vi "PH_Beckhoff_PP_PU.handle PSU DIs.vi"(0 "i ref in":refnum<vi>, 2 "Digital Input Values":T1, 3 "Changed Digital Inputs":i32[](array[numeric]), 5 "error in":errorcluster) -> (14 "i ref out":refnum<vi>, 19 "error out":errorcluster)   [LabVIEW 2014, in "PH_Beckhoff_PP_PU.lvlib"]
uses:
  PH_Beckhoff_PP_PU.lvlib
  PH_Beckhoff/PH_Beckhoff.Digital Inputs.ctl
  PH_Basics/PH_StatusHandler/PH_StatusHandler.lvlib
  PH_Basics/PH_Common/PH_Common.lvlib
  PH_Beckhoff/PH_Beckhoff.lvlib
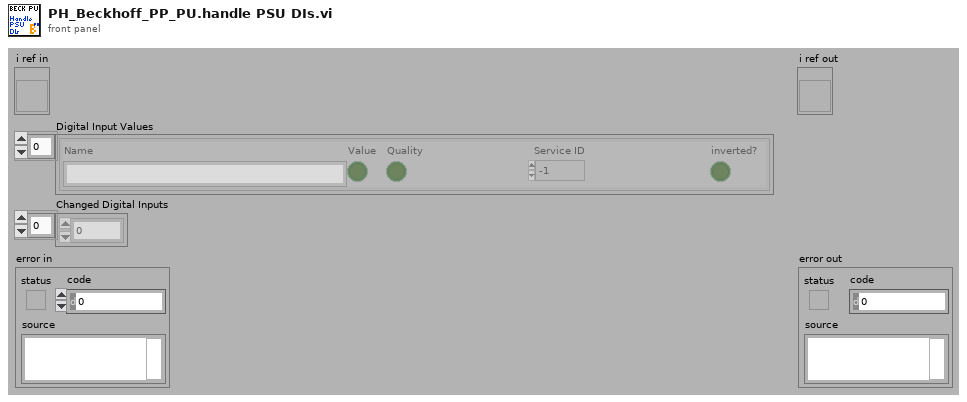
[diagram p1: front panel]
types:
  T1 = typedef "PH_Beckhoff.lvlib/PH_Beckhoff.Digital Inputs.ctl" = cluster{"Name":string, "Value":bool, "Quality":bool, "Service ID":i32, "inverted?":bool}[]
  T2 = typedef "PH_Beckhoff_PP_PU.lvlib/PH_Beckhoff_PP_PU.i attribute.ctl" = cluster{"HV Meas":cluster{"Input GUI Ref":refnum<vi>, "Voltage Service ID":i32, "Voltage [V]":dbl, "Quality":bool, "# in Data":i32}[], "Trigger":cluster{"Status":cluster{"GUI Ref":refnum<vi>, "Status Service ID":i32, "Status":T3}, "last shot:":cluster{"GUI Ref":refnum<vi>, "Service ID":i32, "Time":string}, "DIs":cluster{"triggered":cluster{"GUI Ref":refnum<vi>, "# in Data":i32}, "fired":cluster{"GUI Ref":refnum<vi>, "# in Data":i32}}, "GUI Ref Indicator":refnum<vi>}[], "RR":cluster{"Status":cluster{"GUI Ref":refnum<vi>, "Status Service ID":i32, "Status":T3}, "DIs":cluster{"closed":cluster{"GUI Ref":refnum<vi>, "# in Data":i32}, "open":cluster{"GUI Ref":refnum<vi>, "# in Data":i32}}, "Close":cluster{"GUI Ref":refnum<vi>, "# in Data":i32}, "GUI Ref Indicator":refnum<vi>}[], "Igni":cluster{"Status":cluster{"GUI Ref":refnum<vi>, "Status Service ID":i32, "Status":T3}, "DIs":cluster{"heating on":cluster{"GUI Ref":refnum<vi>, "# in Data":i32}, "water on":cluster{"GUI Ref":refnum<vi>, "# in Data":i32}}, "Device on":cluster{"GUI Ref":refnum<vi>, "# in Data":i32}, "GUI Ref Indicator":refnum<vi>}[], "PSU":cluster{"Status":cluster{"GUI Ref":refnum<vi>, "Status Service ID":i32, "Status":T3}, "Limit Service ID":i32, "DIs":cluster{"inhibit":cluster{"GUI Ref":refnum<vi>, "# in Data":i32}, "end of charge":cluster{"GUI Ref":refnum<vi>, "# in Data":i32}, "HV on":cluster{"GUI Ref":refnum<vi>, "# in Data":i32}, "overtemp":cluster{"GUI Ref":refnum<vi>, "# in Data":i32}, "interlock":cluster{"GUI Ref":refnum<vi>, "# in Data":i32}, "load fault":cluster{"GUI Ref":refnum<vi>, "# in Data":i32}, "sum fault":cluster{"GUI Ref":refnum<vi>, "# in Data":i32}, "HV off":cluster{"GUI Ref":refnum<vi>, "# in Data":i32}, "DC ok":cluster{"GUI Ref":refnum<vi>, "# in Data":i32}}, "AIs":cluster{"voltage":cluster{"GUI Ref":refnum<vi>, "# in Data":i32}, "current":cluster{"GUI Ref":refnum<vi>, "# in Data":i32}}, "DAs":cluster{"inhibit":cluster{"GUI Ref":refnum<vi>, "# in Data":i32}, "interlock":cluster{"GUI Ref":refnum<vi>, "# in Data":i32}, "HV on":cluster{"GUI Ref":refnum<vi>, "# in Data":i32}, "Reset":cluster{"GUI Ref":refnum<vi>, "# in Data":i32}}, "AAs":cluster{"Voltage to set":cluster{"GUI Ref":refnum<vi>, "# in Data":i32}}, "GUI Ref Indicator":refnum<vi>}[], "reconfigured":cluster{"?":bool, "GUI Ref":refnum<vi>}, "PU Rack Type":T4, "HV Meas Info":T5, "PSU Info":T6}
  T3 = typedef "PH_StatusHandler.lvlib/PH_StatusHandler.Status.ctl" = i16
  T4 = typedef "PH_Beckhoff_PP_PU.lvlib/PH_Beckhoff_PP_PU.PU Rack Type.ctl" = enum16{"no Info", "PA 19mm", "PA 45mm", "MA PU 1 and 2", "MA PU 3 and 4", "MA PU 5 and 6", "MA FR and PILC"}
  T5 = typedef "PH_Beckhoff_PP_PU.lvlib/PH_Beckhoff_PP_PU.HV Meas Info.ctl" = cluster{"Period Time [s]":dbl, "Subtractor 1 [Hz]":dbl, "Devider 1 [Hz/kV]":dbl, "Subtractor 2 [Hz]":dbl, "Devider 2 [Hz/kV]":dbl}
  T6 = typedef "PH_Beckhoff_PP_PU.lvlib/PH_Beckhoff_PP_PU.PSU Info.ctl" = cluster{"Limits 1 [V]":cluster{"Lower":dbl, "Upper":dbl}, "Limits 2 [V]":cluster{"Lower":dbl, "Upper":dbl}}
  T7 = cluster{"Status":cluster{"GUI Ref":refnum<vi>, "Status Service ID":i32, "Status":T3}, "Limit Service ID":i32, "DIs":cluster{"inhibit":cluster{"GUI Ref":refnum<vi>, "# in Data":i32}, "end of charge":cluster{"GUI Ref":refnum<vi>, "# in Data":i32}, "HV on":cluster{"GUI Ref":refnum<vi>, "# in Data":i32}, "overtemp":cluster{"GUI Ref":refnum<vi>, "# in Data":i32}, "interlock":cluster{"GUI Ref":refnum<vi>, "# in Data":i32}, "load fault":cluster{"GUI Ref":refnum<vi>, "# in Data":i32}, "sum fault":cluster{"GUI Ref":refnum<vi>, "# in Data":i32}, "HV off":cluster{"GUI Ref":refnum<vi>, "# in Data":i32}, "DC ok":cluster{"GUI Ref":refnum<vi>, "# in Data":i32}}, "AIs":cluster{"voltage":cluster{"GUI Ref":refnum<vi>, "# in Data":i32}, "current":cluster{"GUI Ref":refnum<vi>, "# in Data":i32}}, "DAs":cluster{"inhibit":cluster{"GUI Ref":refnum<vi>, "# in Data":i32}, "interlock":cluster{"GUI Ref":refnum<vi>, "# in Data":i32}, "HV on":cluster{"GUI Ref":refnum<vi>, "# in Data":i32}, "Reset":cluster{"GUI Ref":refnum<vi>, "# in Data":i32}}, "AAs":cluster{"Voltage to set":cluster{"GUI Ref":refnum<vi>, "# in Data":i32}}, "GUI Ref Indicator":refnum<vi>}[]
  T8 = cluster{"Status":cluster{"GUI Ref":refnum<vi>, "Status Service ID":i32, "Status":T3}, "Limit Service ID":i32, "DIs":cluster{"inhibit":cluster{"GUI Ref":refnum<vi>, "# in Data":i32}, "end of charge":cluster{"GUI Ref":refnum<vi>, "# in Data":i32}, "HV on":cluster{"GUI Ref":refnum<vi>, "# in Data":i32}, "overtemp":cluster{"GUI Ref":refnum<vi>, "# in Data":i32}, "interlock":cluster{"GUI Ref":refnum<vi>, "# in Data":i32}, "load fault":cluster{"GUI Ref":refnum<vi>, "# in Data":i32}, "sum fault":cluster{"GUI Ref":refnum<vi>, "# in Data":i32}, "HV off":cluster{"GUI Ref":refnum<vi>, "# in Data":i32}, "DC ok":cluster{"GUI Ref":refnum<vi>, "# in Data":i32}}, "AIs":cluster{"voltage":cluster{"GUI Ref":refnum<vi>, "# in Data":i32}, "current":cluster{"GUI Ref":refnum<vi>, "# in Data":i32}}, "DAs":cluster{"inhibit":cluster{"GUI Ref":refnum<vi>, "# in Data":i32}, "interlock":cluster{"GUI Ref":refnum<vi>, "# in Data":i32}, "HV on":cluster{"GUI Ref":refnum<vi>, "# in Data":i32}, "Reset":cluster{"GUI Ref":refnum<vi>, "# in Data":i32}}, "AAs":cluster{"Voltage to set":cluster{"GUI Ref":refnum<vi>, "# in Data":i32}}, "GUI Ref Indicator":refnum<vi>}
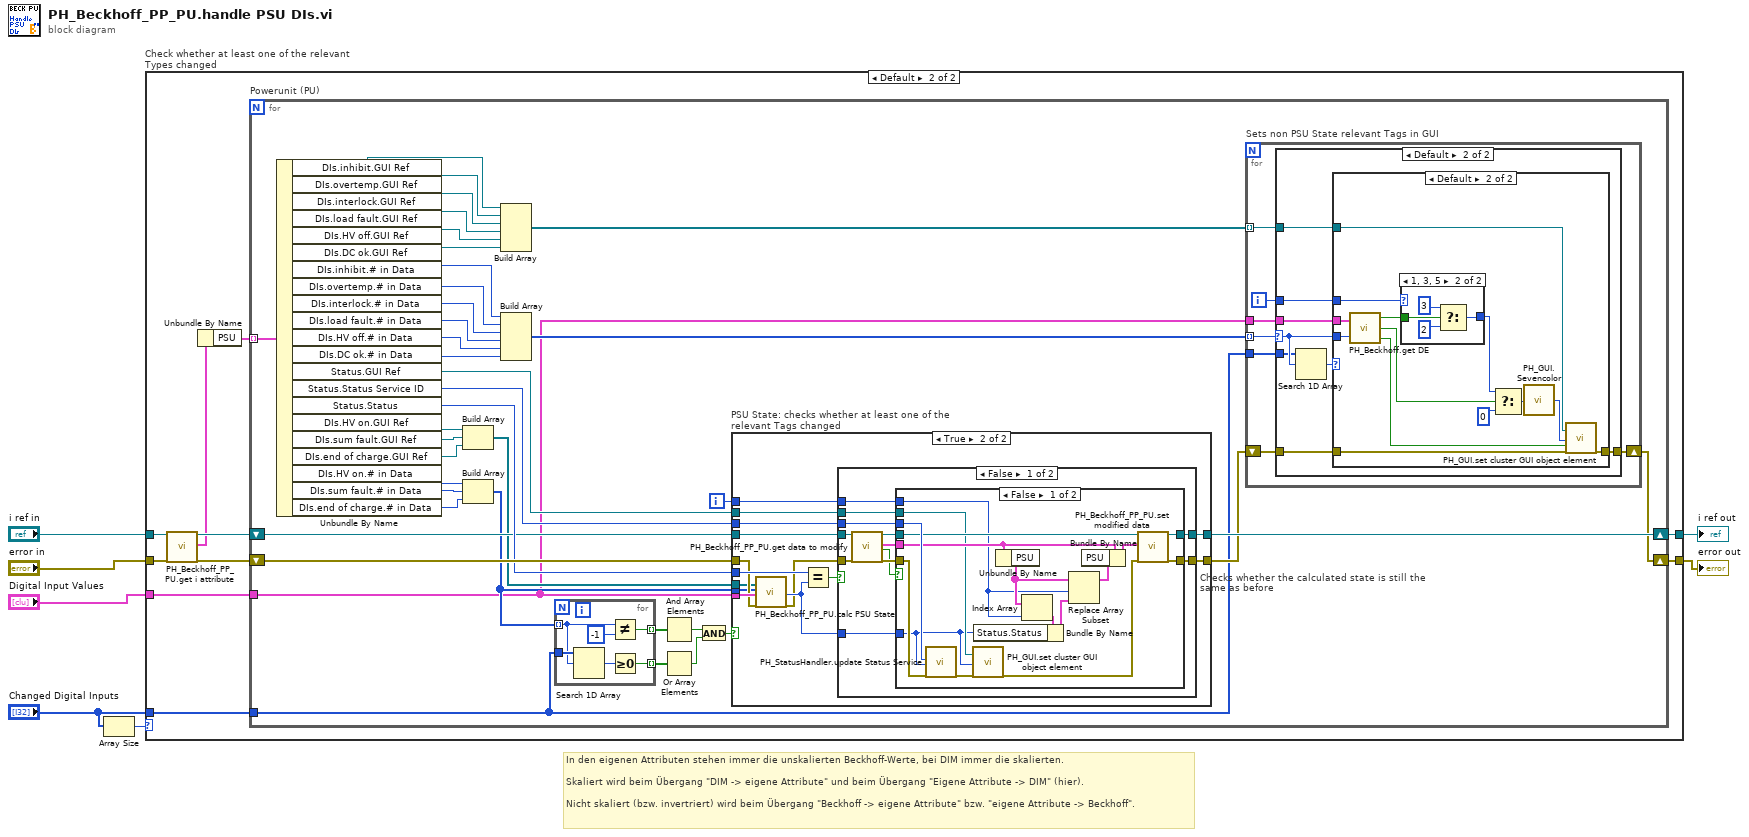
[diagram p0: block diagram]
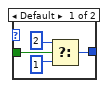
[diagram p5: hidden frame]
diagram:
  # "In den eigenen Attributen stehen immer die unskalierten Beckhoff-Werte, bei DIM immer die skalierten.\n\nSkaliert wird beim Übergang \"DIM -> eigene Attribute\" und beim Übergang \"Eigene Attribute -> DIM\" (hier).\n\nNicht skaliert (bzw. invertriert) wird beim Übergang \"Beckhoff -> eigene Attribute\" bzw. \"eigene Attribute -> Beckhoff\"."
  n1 = Array Size(array="Changed Digital Inputs") -> (size(s)=w2:i32)
  n2 = case "Check whether at least one of the relevant Types changed" shown="Default" w2 {
    tunnel: "i ref in" -> [w9 w15]
    tunnel: "error in" -> [w8 w13]
    tunnel: [w9 w19] -> w6
    tunnel: "Changed Digital Inputs" -> [_ w17]
    tunnel: [w8 w18] -> w7
    tunnel: "Digital Input Values" -> [_ w10]
    frame 0 {
    }
    frame Default {
      n3 = call "PH_Beckhoff_PP_PU.get i attribute.vi"("i ref in"=w15, "error in (no error)"=w13) -> ("i ref out"=w16:refnum<vi>, "i attribute"=w12:T2, "error out"=w14:errorcluster)  [unwired: 15 in]
      n4 = Unbundle By Name(w12) -> ("PSU"=w11:T7)
      n5 = for "Powerunit (PU)" {
        shift-right: [w25] -> w18
        shift-left: w14 -> [w56]
        tunnel: w11 -> [w58] mode=indexing
        shift-right: [w52] -> w19
        shift-left: w16 -> [w54]
        tunnel: w17 -> [w21]
        tunnel: w10 -> [w20]
        i -> [w53]
        n6 = Unbundle By Name(w58) -> ("DIs.inhibit.GUI Ref"=w26:refnum<vi>, "DIs.overtemp.GUI Ref"=w27:refnum<vi>, "DIs.interlock.GUI Ref"=w28:refnum<vi>, "DIs.load fault.GUI Ref"=w29:refnum<vi>, "DIs.HV off.GUI Ref"=w30:refnum<vi>, "DIs.DC ok.GUI Ref"=w37:refnum<vi>, "DIs.inhibit.# in Data"=w31:i32, "DIs.overtemp.# in Data"=w32:i32, "DIs.interlock.# in Data"=w33:i32, "DIs.load fault.# in Data"=w34:i32, "DIs.HV off.# in Data"=w35:i32, "DIs.DC ok.# in Data"=w36:i32, "Status.GUI Ref"=w51:refnum<vi>, "Status.Status Service ID"=w57:i32, "Status.Status"=w55:T3, "DIs.HV on.GUI Ref"=w50:refnum<vi>, "DIs.sum fault.GUI Ref"=w48:refnum<vi>, "DIs.end of charge.GUI Ref"=w49:refnum<vi>, "DIs.HV on.# in Data"=w47:i32, "DIs.sum fault.# in Data"=w45:i32, "DIs.end of charge.# in Data"=w46:i32)
        n7 = Build Array(w50, w48, w49) -> (w38:refnum<vi>[])
        n8 = Build Array(w47, w45, w46) -> (w39:i32[])
        n9 = Build Array(w26, w27, w28, w29, w30, w37) -> (w24:refnum<vi>[])
        n10 = Build Array(w31, w32, w33, w34, w35, w36) -> (w23:i32[])
        n11 = for {
          tunnel: w39 -> [w148] mode=indexing
          tunnel: [w150] -> w44 mode=indexing
          tunnel: w21 -> [w149]
          tunnel: [w145] -> w42 mode=indexing
          n12 = Search 1D Array(1D array=w149, element=w148) -> (index of element=w146:i32)  [unwired: 1 in]
          n13 = Not Equal?(x=w148, y=-1) -> (x != y?=w150:bool)
          n14 = Greater Or Equal To 0?(x=w146) -> (x >= 0?=w145:bool)
        }
        n15 = And Array Elements(Boolean array=w44) -> (logical AND=w43:bool)
        n16 = Or Array Elements(Boolean array=w42) -> (logical OR=w41:bool)
        n17 = And(x=w43, y=w41) -> (x .and. y?=w40:bool)
        n18 = case "PSU State: checks whether at least one of the relevant Tags changed" shown="True" w40 {
          tunnel: w57 -> [_ w112]
          tunnel: w56 -> [w97 w102]
          tunnel: w55 -> [_ w111]
          tunnel: w54 -> [w98 w110]
          tunnel: w53 -> [_ w109]
          tunnel: [w98 w107] -> w52
          tunnel: w20 -> [_ w106]
          tunnel: [w97 w105] -> w22
          tunnel: w51 -> [_ w103]
          tunnel: w39 -> [_ w100]
          tunnel: w38 -> [_ w99]
          frame False {
          }
          frame True {
            n19 = call "PH_Beckhoff_PP_PU.calc PSU State.vi"("GUI Refs: HV on indicator, sum fault and end of charge"=w99, "# in Data: HV on indicator, sum fault and end of charge"=w100, "Digital Inputs"=w106, "error in"=w102) -> ("PSU Status"=w104:T3, "error out"=w101:errorcluster)  [unwired: 14 in]
            n20 = Equal?(x=w111, y=w104) -> (x = y?=w108:bool)
            n21 = case "Checks whether the calculated state is still the same as before" shown="False" w108 {
              tunnel: [w119 w143] -> w105
              tunnel: w112 -> [w124 _]
              tunnel: w101 -> [w123 w143]
              tunnel: w104 -> [w122 _]
              tunnel: w110 -> [w120 w144]
              tunnel: [w117 w144] -> w107
              tunnel: w109 -> [w115 _]
              tunnel: w103 -> [w113 _]
              frame False {
                n22 = call "PH_Beckhoff_PP_PU.get data to modify.vi"("i ref in"=w120, "error in (no error)"=w123) -> ("i ref out"=w118:refnum<vi>, "i attribute"=w116:T2, "timed out"=w114:bool, "error out"=w121:errorcluster)  [unwired: 14 in]
                n23 = case shown="False" w114 {
                  tunnel: w124 -> [w140 _]
                  tunnel: w122 -> [w125 _]
                  tunnel: w121 -> [w139 w141]
                  tunnel: [w138 w141] -> w119
                  tunnel: w118 -> [w137 w142]
                  tunnel: [w136 w142] -> w117
                  tunnel: w116 -> [w135 _]
                  tunnel: w115 -> [w131 _]
                  tunnel: w113 -> [w126 _]
                  frame False {
                    n24 = call "PH_StatusHandler.update Status Service.vi"("Service ID"=w140, "Status"=w125, "error in (no error)"=w139) -> ("error out"=w128:errorcluster)  [unwired: 16 in]
                    n25 = call "PH_GUI.set cluster GUI object element.vi"("Ctl Refnum"=w126, "Value"=w125, "error in"=w128) -> ("error out"=w127:errorcluster)  [unwired: 16 in]
                    n26 = Unbundle By Name(w135) -> ("PSU"=w132:T7)
                    n27 = Index Array(array=w132, index=w131) -> (element=w130:T8)
                    n28 = Bundle By Name(cluster=w130, "Status.Status"=w125) -> (w129:T8)
                    n29 = Replace Array Subset(array=w132, new element=w129, index=w131) -> (w133:T7)
                    n30 = Bundle By Name(cluster=w135, "PSU"=w133) -> (w134:T2)
                    n31 = call "PH_Beckhoff_PP_PU.set modified data.vi"("i ref in"=w137, "i attribute"=w134, "error in (no error)"=w127) -> ("i ref out"=w136:refnum<vi>, "error out"=w138:errorcluster)  [unwired: 15 in]
                  }
                  frame True {
                  }
                }
              }
              frame True {
              }
            }
          }
        }
        n32 = for "Sets non PSU State relevant Tags in GUI" {
          tunnel: w24 -> [w63] mode=indexing
          shift-right: [w65] -> w25
          shift-left: w22 -> [w64]
          tunnel: w23 -> [w60] mode=indexing
          tunnel: w20 -> [w62]
          tunnel: w21 -> [w59]
          i -> [w61]
          n33 = case shown="Default" w60 {
            selector: w60 -> [_ w69]
            tunnel: [w66 w74] -> w65
            tunnel: w64 -> [w66 w73]
            tunnel: w63 -> [_ w72]
            tunnel: w62 -> [_ w71]
            tunnel: w61 -> [_ w70]
            tunnel: w59 -> [_ w68]
            frame -1 {
            }
            frame Default {
              n34 = Search 1D Array(1D array=w68, element=w69) -> (index of element=w67:i32)  [unwired: 1 in]
              n35 = case shown="Default" w67 {
                tunnel: [w75 w88] -> w74
                tunnel: w73 -> [w75 w87]
                tunnel: w72 -> [_ w86]
                tunnel: w71 -> [_ w85]
                tunnel: w70 -> [_ w77]
                tunnel: w69 -> [_ w76]
                frame -1 {
                }
                frame Default {
                  n36 = call "PH_Beckhoff.get DE.vi"("Digital Values"=w85, "index of element"=w76) -> ("Value"=w81:bool, "Quality"=w80:bool, "Tag not found"=w79:bool)
                  n37 = case shown="1, 3, 5" w77 {
                    tunnel: w81 -> [w92 w96]
                    tunnel: [w89 w93] -> w82
                    frame Default {
                      n38 = Select(t=2 ("State"), s=w92, f=1 ("State")) -> (s? t:f=w89:i32)
                    }
                    frame 1, 3, 5 {
                      n39 = Select(t=3 ("State"), s=w96, f=2 ("State")) -> (s? t:f=w93:i32)
                    }
                  }
                  n40 = Select(t=w82, s=w80, f=0 ("State")) -> (s? t:f=w84:i32)
                  n41 = call "PH_GUI.Sevencolor.vi"("State"=w84) -> ("Color Box"=w78:u32)
                  n42 = call "PH_GUI.set cluster GUI object element.vi"("Ctl Refnum"=w86, "Value"=w78, "Blinking? (false)"=w79, "error in"=w87) -> ("error out"=w88:errorcluster)  [unwired: 15 in]
                }
              }
            }
          }
        }
      }
    }
  }
  "error out" <- w7
  "i ref out" <- w6
